vi "GenerateAPIEvent_TopLevel.vi"(6 "Timeout (ms)":u32=600000, 7 "Wait (F)":bool, 8 "error in (no error)":errorcluster, 9 "Task ID":string, 10 "API Command Cluster":T1, 11 "TopLevel in":refnum<class "TopLevel.lvclass">) -> (0 "error out":errorcluster, 3 "TopLevel out":refnum<class "TopLevel.lvclass">)   [LabVIEW 2022 SP3, in "TopLevel.lvclass"]
uses:
  TopLevel.lvclass
  Typedefs/API Command Cluster.ctl
  Typedefs/API Command Enum.ctl
  Typedefs/API Event Data.ctl
  Typedefs/API Task State.ctl
  TopLevel.lvclass/TopLevel.ctl
panel:
  out "Return Value":variant
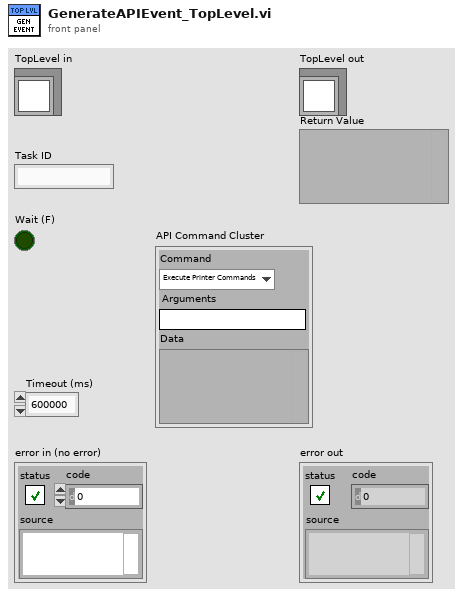
[diagram p1: front panel]
types:
  T1 = typedef "TopLevel.lvclass/API Command Cluster.ctl" = cluster{"Command":T2, "Arguments":string, "Data":variant}
  T2 = typedef "TopLevel.lvclass/API Command Enum.ctl" = enum16{"Execute Printer Commands", "Pre Purge", "Enable Ink Ch-1", "Enable Ink Ch-2", "Enable Ink Ch-3", "Enable Ink Ch-4", "Enable Ink Ch-5", "Enable Ink Ch-6", "Disable Ink Ch-1", "Disable Ink Ch-2", "Disable Ink Ch-3", "Disable Ink Ch-4", "Disable Ink Ch-5", "Disable Ink Ch-6", "ExecuteIdlePrintCycle", "StopIdlePrintCycle", "Abort", "LoadDLP2GUIConfig", "SaveDLP2GUIConfig", "PrimingMode", "SetHeadTemperature", "EnableHead", "EnableHeadHeat", "SetSystemMode", "HeadPrint", "AbortAll", "Send Printer String", "WriteInitXML"}
  T3 = typedef "TopLevel.lvclass/API Task State.ctl" = enum16{"Completed", "Errored", "Pending"}
  T4 = typedef "TopLevel.lvclass/API Event Data.ctl" = cluster{"Task":cluster{"Time Stamp":timestamp, "Timeout (ms)":u32, "Task State":T3, "Task Error":errorcluster, "Task ID":string}, "Command":variant, "Return Value":variant}
  T5 = typedef "TopLevel.lvclass/Private Data.ctl" = cluster{"UserEvents":T6, "All Dependencies":cluster{"Class References":refnum<class>[], "Class Names":string[]}, "Motor Controller Obj":refnum<class "Motor Controller.lvclass">, "IO Obj":refnum<class "IO.lvclass">, "Laser Obj":refnum<class "GIS Printer.lvclass">, "Digilens IPLC Config":T7, "Status":T18, "Database Obj":refnum<class "Database.lvclass">, "DLP2 Obj":refnum<class "DLP2.lvclass">, "MasterConfigurationDLPC2":T19, "DAQ":refnum<class "DAQ.lvclass">, "ConfigDIct":T27, "DLP":T28, "PersistentData":T35, "UserLevel":T36, "ProcessMode":T37, "Str Refnum":refnum<vi>}
  T6 = typedef "TopLevel.lvclass/UserEvents.ctl" = cluster{"API Incoming Event":refnum<user-event>, "API Executed Event":refnum<user-event>, "API Return Event":refnum<user-event>, "Exit Event":refnum<user-event>, "StatusChanged":refnum<user-event>, "DLP GUI Config Changed":refnum<user-event>, "AppEvent":refnum<user-event>, "Login Event":refnum<user-event>, "HeadPrimeStatusEvent":refnum<user-event>}
  T7 = typedef "TopLevel.lvclass/Digilens Config Cluster.ctl" = cluster{"Motion Controller":T8, "IO Config":T9, "PrinterConfiguration":T12, "DAQ Settings":T13}
  T8 = typedef "Motor Controller.lvclass/Motor Controller Config Data.ctl" = cluster{"Motor IP Addresss":string, "Current Position":i32, "Pulse_Per_mm":i32, "PrePrint":dbl[], "Load Position_mm":i32, "Laminate Position_mm":i32}
  T9 = typedef "IO.lvclass/IO Config Data.ctl" = cluster{"DAQDevices":T10[], "DI Channels":T11[], "DO Channels":T11[], "Material Names":string[], "AI Channels":T11[], "AO Channels":T11[]}
  T10 = typedef "IO.lvclass/DCON_DeviceConfig--Cluster.ctl" = cluster{"COM":string, "DeviceName":string, "BaudRate":u32, "Number of Channels":i32, "DeviceAddress":i32, "Enable":bool}
  T11 = typedef "IO.lvclass/Channel Data.ctl" = cluster{"Channel Name":string, "Device Name":string, "Channel No":string}
  T12 = typedef "GIS Printer.lvclass/PrinterConfiguration--Cluster.ctl" = cluster{"IPAddress":string, "Move Stage on RTP Command?":bool, "Stage Move Position":string, "PH1-Prime Path":path, "PH2-Prime Path":path, "PH3-Prime Path":path, "PH4-Prime Path":path, "PH5-Prime Path":path, "PH6-Prime Path":path, "PrintScriptsFolder":path, "PurgeScriptsFolder":path, "StageScriptsFolder":path, "PH1-HeatOn Path":path, "PH2-HeatOn Path":path, "PH3-HeatOn Path":path, "PH4-HeatOn Path":path, "PH5-HeatOn Path":path, "PH6-HeatOn Path":path, "PH1-HeatOff Path":path, "PH2-HeatOff Path":path, "PH3-HeatOff Path":path, "PH4-HeatOff Path":path, "PH5-HeatOff Path":path, "PH6-HeatOff Path":path}
  T13 = typedef "DAQ.lvclass/TD DAQ Settings--cluster.ctl" = cluster{"Simulate DAQ":bool, "DI Settings":T14[], "AI Settings":T15[], "Relay IONames":string[], "AO IONames":string[], "AO NChan SingleTask":bool}
  T14 = typedef "DAQ.lvclass/TD DI Instrument Settings--cluster.ctl" = cluster{"Disable":bool, "DI TaskName":string, "DI RefreshIntv":i32}
  T15 = typedef "DAQ.lvclass/TD AI Instrument Settings--cluster.ctl" = cluster{"Disable":bool, "AI TaskName":string, "AI InstSettings":T16, "SimAI Ranges":T17}
  T16 = typedef "DAQ.lvclass/TD AI InstSettings--cluster.ctl" = cluster{"DaqRate":dbl, "NumSamples":i32}
  T17 = typedef "DAQ.lvclass/TD SimAI Ranges--cluster.ctl" = cluster{"lo":dbl, "hi":dbl}
  T18 = typedef "Status_TopLevel--Cluster.ctl" = cluster{"Busy":bool, "Time":timestamp, "error":errorcluster, "PrintNo":i32, "PrePurgePrintNo":i32, "CalPrintNo":i32}
  T19 = typedef "TD MasterConfiguration DLPC2--cluster.ctl" = cluster{"Paths":T20, "ColorPaneMapping":T21, "Materials":string[], "ColorPlanes":string[], "SpitVoltages_Half":T23, "SpitVoltages_Full":T23, "SystemMode":string[], "PrimeModeConfig":T24[], "Running Average Duration_s":dbl}
  T20 = typedef "DLPC2_Path--Cluster.ctl" = cluster{"DigiBit WG Design Folder":path, "Compensated GS Image Folder":path, "Nozzle GS Files Head 1":path, "Nozzle GS Files Head 2":path, "Nozzle GS Files Head 3":path, "Nozzle GS Files Head 4":path, "Nozzle GS Files Head 5":path, "Nozzle GS Files Head 6":path}
  T21 = typedef "TD HeadColorPaneMappingAll--cluster.ctl" = cluster{"Head 1":T22, "Head 2":T22, "Head 3":T22, "Head 4":T22, "Head 5":T22, "Head 6":T22}
  T22 = typedef "TD HeadColorPaneMapping--cluster.ctl" = cluster{"Material":string, "ColorPane":string}
  T23 = typedef "SpitVoltages--Cluster.ctl" = cluster{"1":dbl, "2":dbl, "3":dbl, "4":dbl, "5":dbl, "6":dbl}
  T24 = typedef "TopLevel.lvclass/PrimingMode APIData.ctl" = cluster{"Interval (s)":dbl, "PurgeDuration (s)":dbl, "Repeats":u8, "PrimingMode":T25, "Head":T26, "Frequency (Hz)":i32, "PrintWeight":dbl}
  T25 = typedef "PurgeMode--Enum.ctl" = enum16{"Pre-Purge", "Purge", "Spit", "Shake"}
  T26 = typedef "PrinterHeads--Enum.ctl" = enum16{"-1", "1", "2", "3", "4", "5", "6"}
  T27 = typedef "TD Dynamic CVT DVR--ref.ctl" = refnum<data-value>
  T28 = typedef "DLPConfig_Initialization.ctl" = cluster{"PrinterInitialization":cluster{"Printer":cluster{"#attributes":cluster{"Name":string}}, "VacPumpSet":cluster{"#attributes":cluster{"VacPumpEnable":bool, "VacPumpSpeed":dbl}}, "HIBEnable":cluster{"#attributes":cluster{"HIB1Enable":bool, "HIB2Enable":bool, "HIB3Enable":bool, "HIB4Enable":bool, "HIB5Enable":bool, "HIB6Enable":bool}}, "PrinterCompensation":T29}, "HeadSet":cluster{"HeadProperties":T30[]}, "InkSet":cluster{"Ink":T32[]}, "Troubleshooting":cluster{"PMBLogging":cluster{"#attributes":cluster{"PMBMonitorDuringPrint":bool, "PMBMonitorDuringIdle":bool, "LogSwatheInputData":bool, "LogSwatheOutputData":bool, "LogPrintheadColourPlanes":bool, "LogPMBCommunication":bool, "LogSimulatedOutput":bool, "LogAllPMBCommunicationData":bool, "LogPMBSpace":bool, "ExtendedPMBSpaceLogging":bool, "LogPMBWriteSpeed":bool, "LogUsbRetries":bool}}, "HIBLogging":cluster{"#attributes":cluster{"HIBMonitoringDuringPrint":bool, "HIBMonitoringLog":bool}}}}
  T29 = typedef "DLP2_PrinterCompensationProperties.ctl" = cluster{"#attributes":cluster{"AppName":string, "PrintWeightMultiplier":dbl, "Rotation":bool, "Driver":string, "Server":string, "Database":string, "User":string, "Password":string}}
  T30 = typedef "DLP2_PrinterHeadProperties.ctl" = cluster{"#attributes":T31}
  T31 = typedef "DLPConfig)Init_HeadPropertyAttr--Cluster.ctl" = cluster{"HeadNumber":u8, "Material":string, "HeadLocalX":dbl, "HeadLocalY":dbl, "HeadRotationAngle":dbl, "VH2L_Hi":dbl, "VH2R_Hi":dbl, "VH1LA_Hi":dbl, "VH1LB_Hi":dbl, "VH1RA_Hi":dbl, "VH1RB_Hi":dbl, "VH2L_Lo":dbl, "VH2R_Lo":dbl, "VH1LA_Lo":dbl, "VH1LB_Lo":dbl, "VH1RA_Lo":dbl, "VH1RB_Lo":dbl}
  T32 = typedef "DLP2_PrinterMaterialProperties.ctl" = cluster{"#attributes":cluster{"InkType":string, "PrePrintPurge":bool, "PurgeTime":dbl, "PurgeCount":i32, "Density":dbl, "NumberofDrops":i32, "PrintWeight":dbl, "PrintheadPrime":bool}, "Idle":T33, "Process":T34}
  T33 = typedef "InkIdleNodeConfigXML--Cluster.ctl" = cluster{"ShortIdle":cluster{"#attributes":cluster{"Heat":dbl, "Meniscus":dbl, "Recirculation":bool}}, "LongIdle":cluster{"#attributes":cluster{"Heat":dbl, "Meniscus":dbl, "Recirculation":bool}}}
  T34 = typedef "InkProcessNodeConfigXML--Cluster.ctl" = cluster{"C30_Process":cluster{"#attributes":cluster{"Heat":dbl, "Meniscus":dbl, "Recirculation":bool, "ColorPlane":string}}, "S30_Process":cluster{"#attributes":cluster{"Heat":dbl, "Meniscus":dbl, "Recirculation":bool, "ColorPlane":string}}}
  T35 = typedef "PersistentData--Cluster.ctl" = cluster{"ToolIdle":bool, "Meniscus Vac Pump Speed":dbl, "InkChEnable":cluster{"Enable Ink Ch-1":bool, "Enable Ink Ch-2":bool, "Enable Ink Ch-3":bool, "Enable Ink Ch-4":bool, "Enable Ink Ch-5":bool, "Enable Ink Ch-6":bool}, "HeatEnable":cluster{"Heater-1 Off":bool, "Heater-2 Off":bool, "Heater-3 Off":bool, "Heater-4 Off":bool, "Heater-5 Off":bool, "Heater-6 Off":bool}, "MiniscusPressure":cluster{"Meniscus Pressure Set - R1":dbl, "Meniscus Pressure Set - R2":dbl, "Meniscus Pressure Set - R3":dbl, "Meniscus Pressure Set - R4":dbl, "Meniscus Pressure Set - R5":dbl, "Meniscus Pressure Set - R6":dbl}, "RecircPumpFlow":cluster{"Recirc Pump Flow Set - R1":dbl, "Recirc Pump Flow Set - R2":dbl, "Recirc Pump Flow Set - R3":dbl, "Recirc Pump Flow Set - R4":dbl, "Recirc Pump Flow Set - R5":dbl, "Recirc Pump Flow Set - R6":dbl}}
  T36 = typedef "UserLevel--Enum.ctl" = enum16{"None", "Operator", "Engineer"}
  T37 = typedef "processMode--enum.ctl" = enum16{"Short Idle", "Long Idle ", "C30_Process", "S30_Process"}
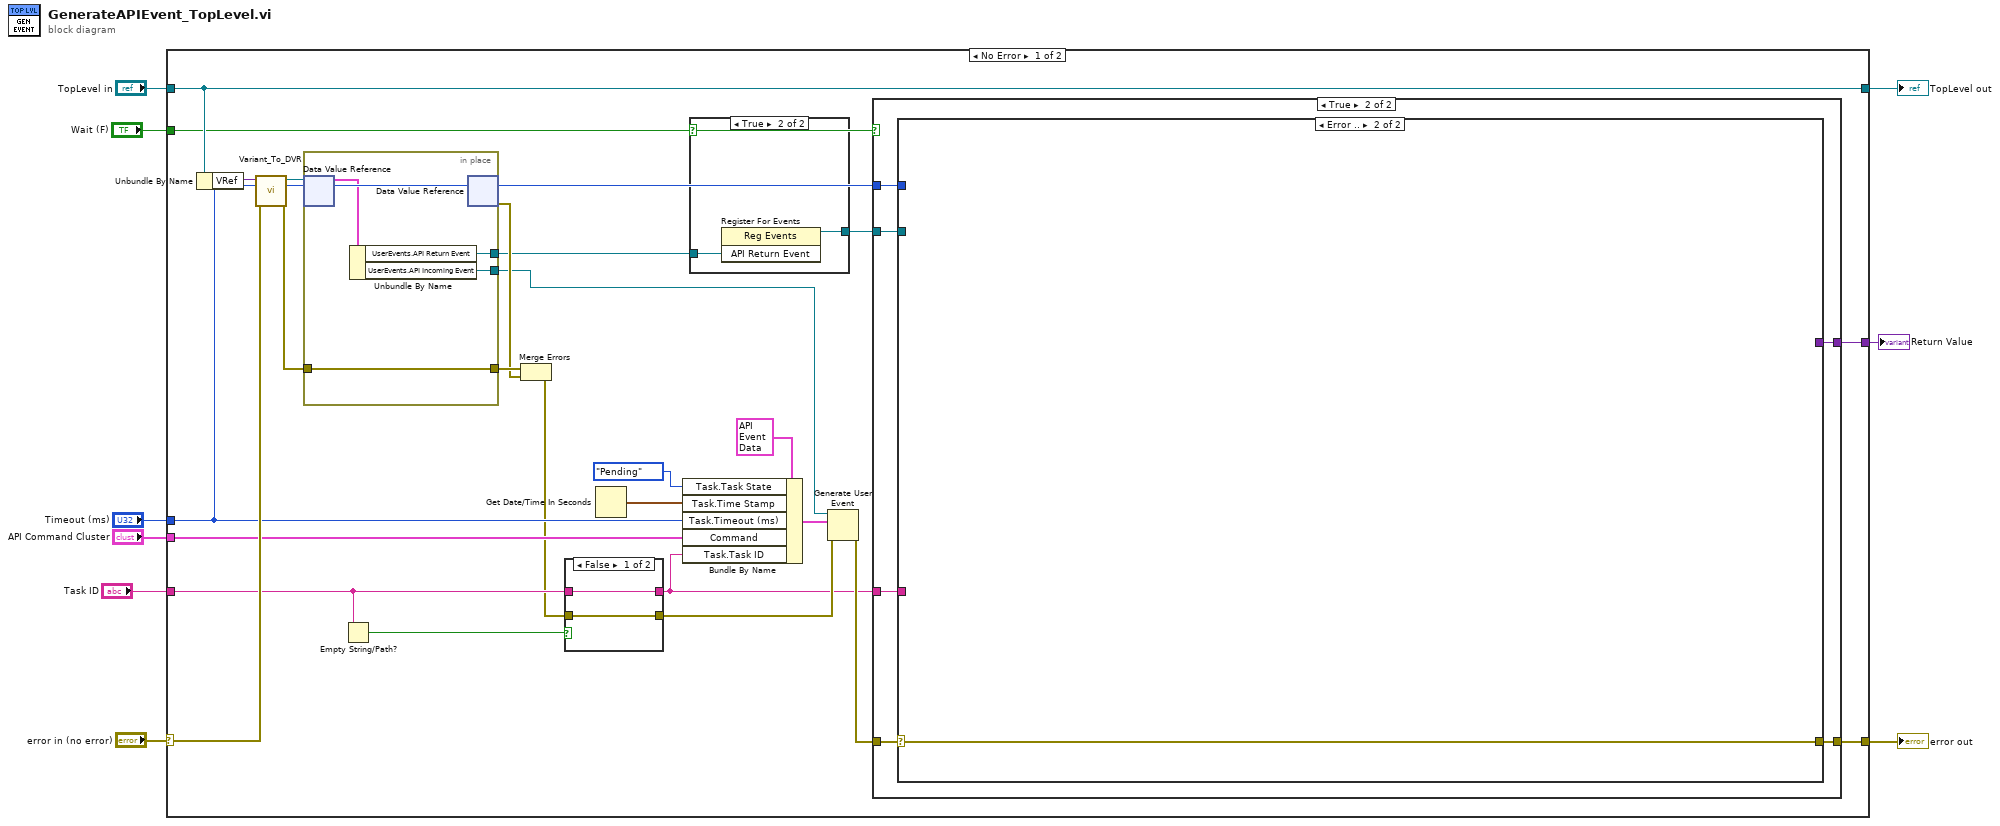
[diagram p0: block diagram]
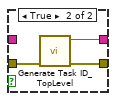
[diagram p2: hidden frame]
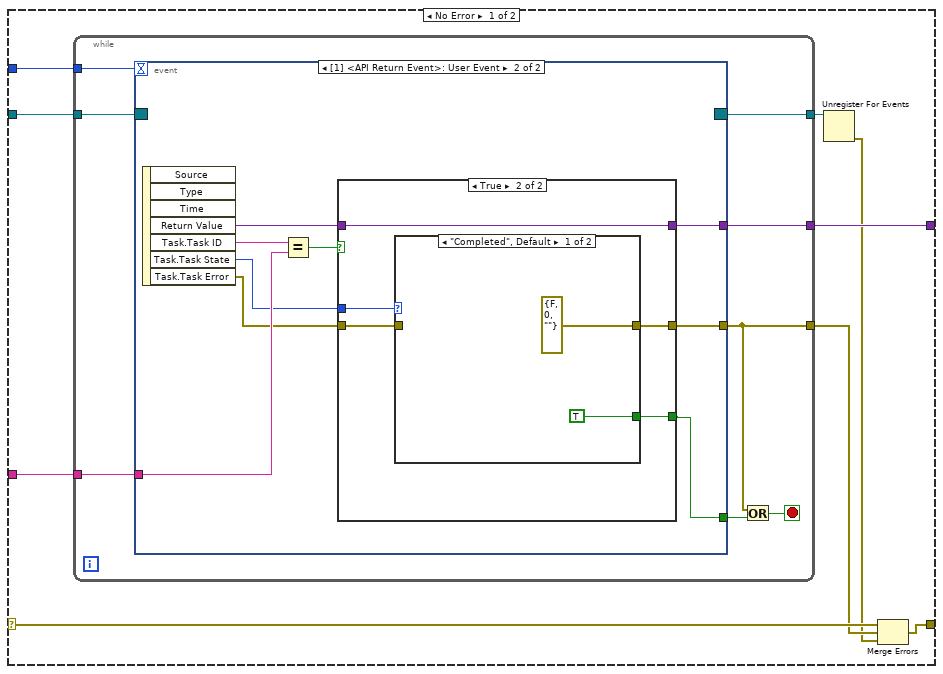
[diagram p4: hidden frame]
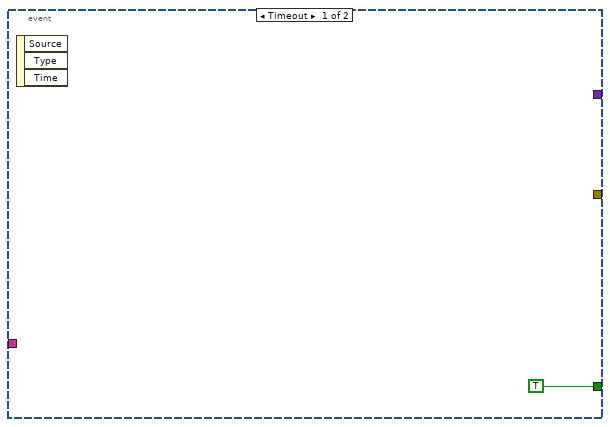
[diagram p5: hidden frame]
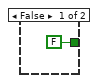
[diagram p6: hidden frame]
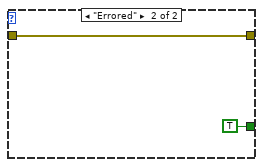
[diagram p7: hidden frame]
diagram:
  n1 = case shown="No Error" "error in (no error)" {
    selector: "error in (no error)" -> [w34 w92]
    tunnel: [w15 w92] -> w8
    tunnel: [w28 w91] -> w6
    tunnel: "TopLevel in" -> [w28 w91]
    tunnel: "Wait (F)" -> [w21 _]
    tunnel: "Timeout (ms)" -> [w19 _]
    tunnel: "API Command Cluster" -> [w22 _]
    tunnel: [w16 _] -> w2
    tunnel: "Task ID" -> [w13 _]
    frame No Error {
      n2 = Unbundle By Name(w28) -> ("VRef"=w33:variant)
      n3 = call "Variant_To_DVR.vi"("error in (no error)"=w34, "Variant"=w33) -> ("error out"=w31:errorcluster, "DVR"=w32:refnum<data-value>)  [unwired: 8 in]
      n4 = in-place {
        in-place-border: w31 -> [w89]
        in-place-border: [w89] -> w30
        in-place-border: [w88] -> w27
        in-place-border: [w87] -> w26
        n5 = in-place-dvr #1(w32) -> (w90:T5)  [unwired: 1 out]
        n6 = Unbundle By Name(w90) -> ("UserEvents.API Return Event"=w88:refnum<user-event>, "UserEvents.API Incoming Event"=w87:refnum<user-event>)
        n7 = in-place-dvr #1() -> (w29:errorcluster)  [unwired: 1 in, 1 out]
      }
      n8 = Empty String/Path?(string/path=w13) -> (empty?=w14:bool)
      n9 = Merge Errors(w30, w29) -> (w12:errorcluster)
      n10 = case shown="False" w14 {
        tunnel: [w36 w39] -> w10
        tunnel: w13 -> [w36 _]
        tunnel: w12 -> [w35 w38]
        tunnel: [w35 w37] -> w11
        frame False {
        }
        frame True {
          n11 = call "Generate Task ID_TopLevel.vi"("error in (no error)"=w38) -> ("error out"=w37:errorcluster, "Task ID"=w39:string)  [unwired: 9 in]
        }
      }
      n12 = Get Date/Time In Seconds() -> (seconds since 1Jan1904=w24:timestamp)
      n13 = Bundle By Name(cluster=T4 {"Task"={"Time Stamp"=timestamp(0 s since 1904-01-01), "Timeout (ms)"=0, "Task State"=enum."Completed", "Task Error"={"status"=FALSE, "code"=0, "source"=""}, "Task ID"=""}, "Command"=variant, "Return Value"=variant} ("event data"), "Task.Task State"=API_Task_State."Pending", "Task.Time Stamp"=w24, "Task.Timeout (ms)"=w19, "Command"=w22, "Task.Task ID"=w10) -> (w23:T4)
      n14 = case shown="True" w21 {
        tunnel: w27 -> [_ w86]
        tunnel: [_ w85] -> w18
        frame False {
        }
        frame True {
          n15 = register-events(w86) -> (reference out=w85:refnum<event-registration>)  [unwired: 2 in, 1 out]
        }
      }
      n16 = Generate User Event(user event=w26, event data cluster=w23, error in=w11) -> (error out=w20:errorcluster)  [unwired: 1 in, 1 out]
      n17 = case shown="True" w21 {
        tunnel: w20 -> [w40 w46]
        tunnel: w19 -> [_ w45]
        tunnel: w18 -> [_ w44]
        tunnel: [_ w43] -> w16
        tunnel: [w40 w42] -> w15
        tunnel: w10 -> [_ w41]
        frame False {
        }
        frame True {
          n18 = case shown="Error .." w46 {
            selector: w46 -> [w51 w84]
            tunnel: w45 -> [w55 _]
            tunnel: w44 -> [w54 _]
            tunnel: [w53 _] -> w43
            tunnel: [w48 w84] -> w42
            tunnel: w41 -> [w47 _]
            frame No Error {
              n19 = while {
                tunnel: w55 -> [w63]
                tunnel: w54 -> [w62]
                tunnel: [w61] -> w53
                tunnel: [w58] -> w52
                tunnel: [w57] -> w50
                tunnel: w47 -> [w56]
                stop <- w59 stop-if-true
                n20 = event shown="[1] <API Return Event>: User Event" {
                  selector: w62 -> [_ _]
                  dyn-events: [_ _] -> w58
                  timeout: w63 -> [_ _]
                  tunnel: [_ w67] -> w61
                  tunnel: [_ w66] -> w57
                  tunnel: [TRUE w65] -> w60
                  tunnel: w56 -> [_ w72]
                  event Timeout {
                    n21 = event-data() -> ()  [unwired: 1 in, 3 out]
                  }
                  event User Event {
                    n22 = event-data() -> ("Return Value"=w71:variant, "Task.Task ID"=w73:string, "Task.Task State"=w69:T3, "Task.Task Error"=w68:errorcluster)  [unwired: 1 in, 3 out]
                    n23 = Equal?(x=w73, y=w72) -> (x = y?=w70:bool)
                    n24 = case shown="True" w70 {
                      tunnel: w69 -> [_ w79]
                      tunnel: w68 -> [_ w78]
                      tunnel: [_ w77] -> w67
                      tunnel: w71 -> [_ w77]
                      tunnel: [_ w76] -> w66
                      tunnel: [FALSE w75] -> w65
                      frame False {
                      }
                      frame True {
                        n25 = case shown="\"Completed\", Default" w79 {
                          tunnel: w78 -> [_ w83]
                          tunnel: [errorcluster {"status"=FALSE, "code"=0, "source"=""} ("Task Error") w83] -> w76
                          tunnel: [TRUE TRUE] -> w75
                          frame "Completed", Default {
                          }
                          frame "Errored" {
                          }
                        }
                      }
                    }
                  }
                }
                n26 = Or(x=w57, y=w60) -> (x .or. y?=w59:bool)
              }
              n27 = Unregister For Events(event registration refnum=w52) -> (error out=w49:errorcluster)  [unwired: 1 in]
              n28 = Merge Errors(w51, w50, w49) -> (w48:errorcluster)
            }
            frame Error {
            }
          }
        }
      }
    }
    frame Error {
    }
  }
  "error out" <- w8
  "TopLevel out" <- w6
  "Return Value" <- w2
